vi "DataGraph_ShortcutMenu.vi"(7 "ShortCut Menu Enable":bool, 8 "error in (no error)":errorcluster, 11 "menu reference":refnum<k9>) -> (0 "error out":errorcluster, 3 "menu reference out":refnum<k9>)   [LabVIEW 2018, in "DataGraphXControl.xctl"]
uses:
  DataGraphXControl.xctl
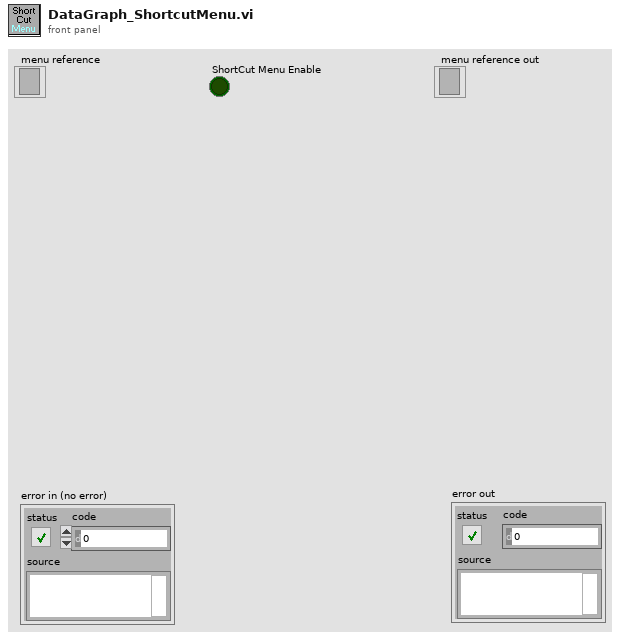
[diagram p1: front panel]
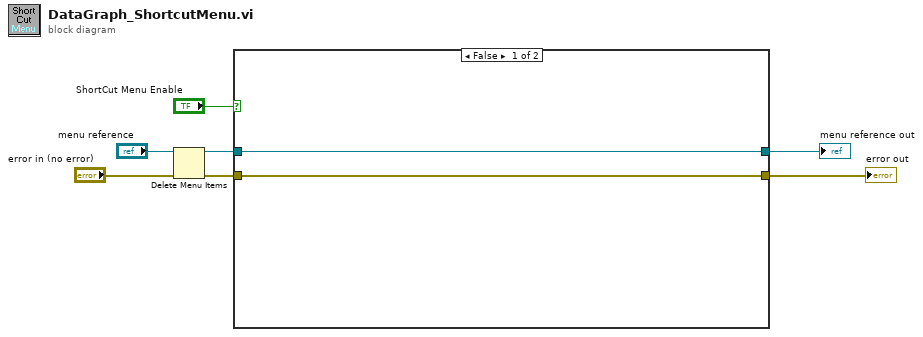
[diagram p0: block diagram]
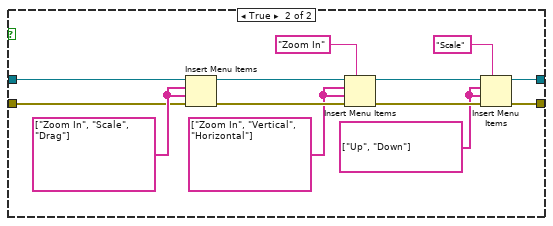
[diagram p2: hidden frame]
diagram:
  n1 = Delete Menu Items(6:"error in (no error)", 9:"menu reference") -> (0:w4:errorcluster, 3:w7:refnum<k9>)  [unwired: 2 in]
  n2 = case shown="False" "ShortCut Menu Enable" {
    tunnel: w7 -> [w9 w22]
    tunnel: [w9 w12] -> w5
    tunnel: w4 -> [w8 w11]
    tunnel: [w8 w10] -> w3
    frame False {
    }
    frame True {
      w13 = string[] ["Up", "Down"] ("item tags")
      w17 = string[] ["Zoom In", "Vertical", "Horizontal"] ("item tags")
      w19 = string[] ["Zoom In", "Scale", "Drag"] ("item tags")
      n3 = Insert Menu Items(6:w11, 7:w19, 8:w19, 9:w22) -> (0:w20:errorcluster, 3:w21:refnum<k9>)  [unwired: 2 in, 1 out]
      n4 = Insert Menu Items(5:"Zoom In", 6:w20, 7:w17, 8:w17, 9:w21) -> (0:w15:errorcluster, 3:w16:refnum<k9>)  [unwired: 1 in, 1 out]
      n5 = Insert Menu Items(5:"Scale" ("menu tag"), 6:w15, 7:w13, 8:w13, 9:w16) -> (0:w10:errorcluster, 3:w12:refnum<k9>)  [unwired: 1 in, 1 out]
    }
  }
  "menu reference out" <- w5
  "error out" <- w3
